vi "Convert selected data to Fluofit.vi"() -> ()   [LabVIEW 2009]
uses:
  <vilib>/Utility/file.llb/Read From Spreadsheet File (DBL).vi
panel:
  out "path names":path[](array[path])
  in  "name format":u16(ring) items=["#.xml_decay of spotxxx.dat", "#_decay of spotxxx.dat"]
  in  "string to append":string="_selected_spots_decays.txt"
  out "output path of created file":path
  in  "selection path":path=path "V:/Tinnefeld/Data/waveguides/20110512 Auswertung/20110427_nochmal/7L/2"
  out "appended array":dbl[][](array[numeric])
  in  "channel of interest":i32=7
  out "all rows":dbl[][](array[numeric]) format="%0.3f"
  # "Merges chosen channel (=row in data file, specified below)\ninto one *.dat file\nChoose selected results file from\"result screener\"\nand all corresponding *.dat files are merged for fluofit\nfirst column: time\nall other columns: decays of interest\n\nplease use the following terminology\n\n/2/2_decay of spot000.dat \n/2/2_decay of spot001.dat\n...\n/3\n...\n/4\n...\nselected_results.txt (name of this file doesn't matter, but must be in this folder)\n\nfolder and spot names don't need to be numbered in increments,\nbut have to be numbers!"
  # "IMPORTANT part : -->"
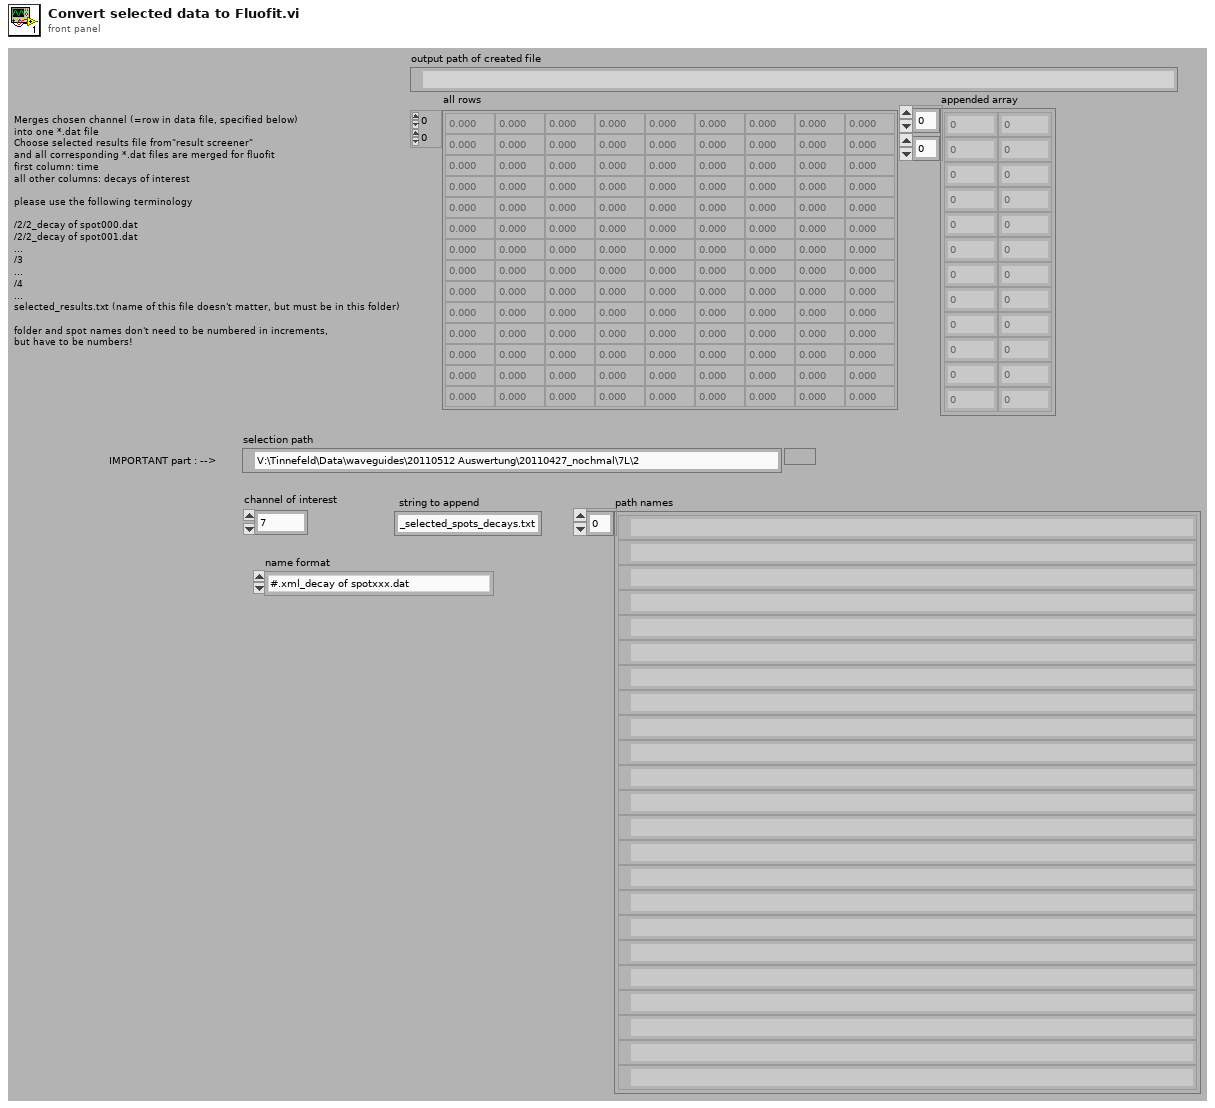
[diagram p1: front panel]
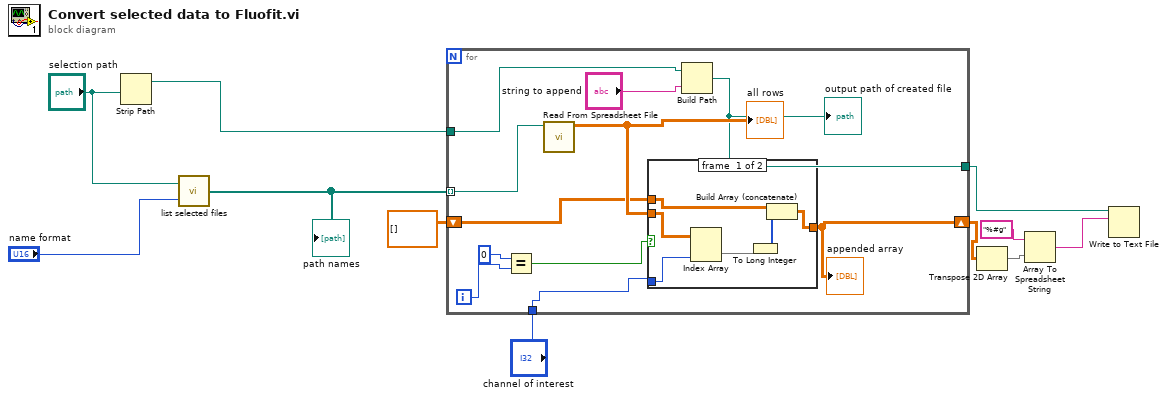
[diagram p0: block diagram]
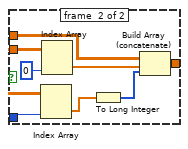
[diagram p2: hidden frame]
diagram:
  n1 = Strip Path(path="selection path") -> (stripped path=w5:path)  [unwired: 1 out]
  n2 = call "list selected files.vi"("Ring"="name format", "selection path"="selection path") -> ("path names"=w3:path[])
  "path names" <- w3
  n3 = for {
    tunnel: "channel of interest" -> [w21]
    tunnel: w5 -> [w13]
    tunnel: [w12] -> w2
    shift-right: [w19] -> w9
    shift-left: dbl[][] [] -> [w20]
    tunnel: w3 -> [w15] mode=indexing
    i -> [w18]
    n4 = Equal?(x=0, y=w18) -> (x = y?=w16:bool)
    n5 = call-poly <vilib>:"Read From Spreadsheet File.vi"("file path (dialog if empty)"=w15) -> ("all rows"=w22:dbl[][])  [unwired: 6 in, 4 out]
    "all rows" <- w22
    n6 = case shown="False" w16 {
      tunnel: w22 -> [w27 w35]
      tunnel: w21 -> [w28 w33]
      tunnel: w20 -> [w24 w32]
      tunnel: [w25 w31] -> w19
      frame #0 {
        n7 = Index Array(array=w27, index (col)=w28) -> (element=w26:dbl[])  [unwired: 1 in]
        n8 = To Long Integer(number=w26) -> (32bit integer=w23:i32[])
        n9 = Build Array (concatenate)(w24, w23) -> (w25:dbl[][])
      }
      frame #1 {
        n10 = Index Array(array=w35, index (col)=w33) -> (element=w30:dbl[])  [unwired: 1 in]
        n11 = Index Array(array=w35, index (col)=0 ("disabled index (col)")) -> (element=w36:dbl[])  [unwired: 1 in]
        n12 = To Long Integer(number=w30) -> (32bit integer=w29:i32[])
        n13 = Build Array (concatenate)(w32, w36, w29) -> (w31:dbl[][])
      }
    }
    "appended array" <- w19
    n14 = Build Path(base path=w13, name or relative path="string to append") -> (appended path=w12:path)
    "output path of created file" <- w12
  }
  n15 = Transpose 2D Array(2D array=w9) -> (transposed array=w7:dbl[][])
  n16 = Array To Spreadsheet String(array=w7, 3:"%#g" ("format string")) -> (spreadsheet string=w6:string)  [unwired: 1 in]
  n17 = Write to Text File(file (use dialog)=w2, text=w6) -> ()  [unwired: 2 in, 3 out]
